vi "OAT Tachless Add Control Point_sub.vi"(10 "New Control Point":cluster{dbl, dbl} {"?" format="%.2f"; "?" format="%.2f"}, 11 "Control Points":cluster{"X":dbl[], "Y":dbl[]} {"Y" format="%.2f"; "X" format="%.2f"}) -> (3 "Control Points Out":cluster{"X":dbl[], "Y":dbl[]} {"Y" format="%.2f"; "X" format="%.2f"})   [LabVIEW 2017, in "SoundVib_Tachless.lvlib"]
uses:
  <vilib>/addons/Sound and Vibration/Order Analysis/Tachless/SoundVib_Tachless.lvlib
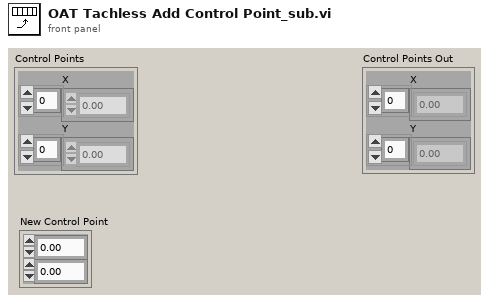
[diagram p1: front panel]
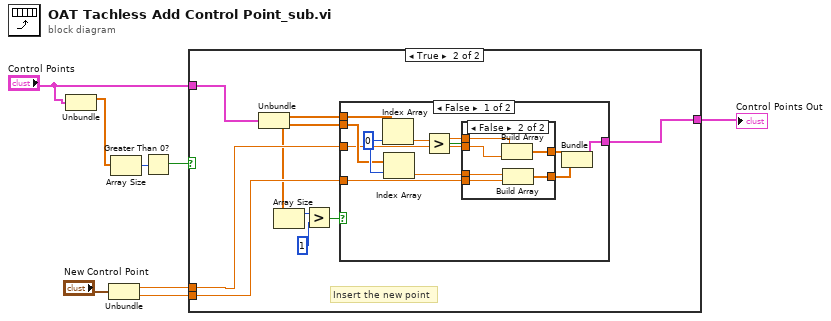
[diagram p0: block diagram]
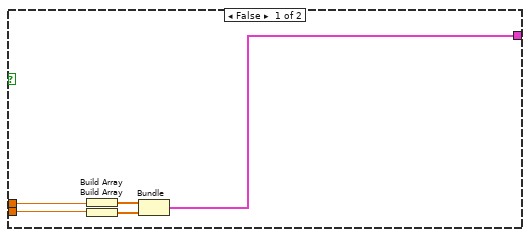
[diagram p2: hidden frame]
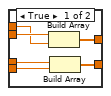
[diagram p3: hidden frame]
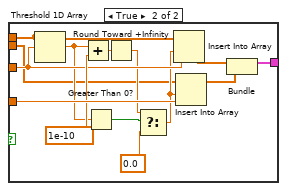
[diagram p4: hidden frame]
diagram:
  n1 = Unbundle("Control Points") -> ("X"=w3:dbl[])  [unwired: 1 out]
  n2 = Unbundle("New Control Point") -> (w6:dbl, w8:dbl)
  n3 = Array Size(array=w3) -> (size(s)=w5:i32)
  n4 = Greater Than 0?(x=w5) -> (x > 0?=w4:bool)
  n5 = case shown="True" w4 {
    tunnel: w8 -> [w12 w22]
    tunnel: w6 -> [w13 w20]
    tunnel: [w9 w14] -> w2
    tunnel: "Control Points" -> [_ w15]
    frame False {
      n6 = Build Array(w13) -> (w11:dbl[])
      n7 = Build Array(w12) -> (w10:dbl[])
      n8 = Bundle(w11, w10) -> (w9:cluster{dbl[], dbl[]})  [unwired: 1 in]
    }
    frame True {
      # "Insert the new point"
      n9 = Unbundle(w15) -> ("X"=w21:dbl[], "Y"=w19:dbl[])
      n10 = Array Size(array=w19) -> (size(s)=w17:i32)
      n11 = Greater?(x=w17, y=1) -> (0:w18:bool)
      n12 = case shown="False" w18 {
        tunnel: w22 -> [w27 w59]
        tunnel: w21 -> [w33 w58]
        tunnel: [w23 w55] -> w14
        tunnel: w20 -> [w26 w52]
        tunnel: w19 -> [w29 w47]
        frame False {
          w30 = 0 ("Index")
          n13 = Index Array(array=w33, index=w30) -> (element=w32:dbl)
          n14 = Index Array(array=w29, index=w30) -> (element=w28:dbl)
          n15 = Greater?(x=w32, y=w26) -> (0:w31:bool)
          n16 = case shown="False" w31 {
            tunnel: w32 -> [w38 w42]
            tunnel: w28 -> [w37 w41]
            tunnel: w27 -> [w36 w40]
            tunnel: [w35 w45] -> w25
            tunnel: [w34 w44] -> w24
            tunnel: w26 -> [w39 w43]
            frame True {
              n17 = Build Array(w39, w38) -> (w35:dbl[])
              n18 = Build Array(w36, w37) -> (w34:dbl[])
            }
            frame False {
              n19 = Build Array(w42, w43) -> (w45:dbl[])
              n20 = Build Array(w41, w40) -> (w44:dbl[])
            }
          }
          n21 = Bundle(w25, w24) -> (w23:cluster{dbl[], dbl[]})  [unwired: 1 in]
        }
        frame True {
          n22 = Threshold 1D Array(2:w52, 3:w58) -> (0:w51:dbl)  [unwired: 1 in]
          n23 = Add(x=w51, y=1e-10) -> (x+y=w54:dbl)
          n24 = Greater Than 0?(x=w51) -> (x > 0?=w46:bool)
          n25 = Round Toward +Infinity(x=w54) -> (ceil(x): smallest int >= x=w50:dbl)
          n26 = Select(t=w50, s=w46, f=0.0) -> (s? t:f=w48:dbl)
          n27 = Insert Into Array(array=w58, index=w48, new element=w52) -> (w57:dbl[])
          n28 = Insert Into Array(array=w47, index=w48, new element=w59) -> (w56:dbl[])
          n29 = Bundle("X"=w57, "Y"=w56) -> (w55:cluster{"X":dbl[], "Y":dbl[]})  [unwired: 1 in]
        }
      }
    }
  }
  "Control Points Out" <- w2
